vi "byte available write serial.vi"(11 "resourceId":i32) -> (2 "byte available":i32, 3 "resourceId out":i32)   [LabVIEW 2010, in "libcommon_serial.lvlib"]
doc: "int byte_available_write_serial(pserial_handle_t h);"
uses:
  <userlib>/libcommon_serial/libcommon_serial.lvlib
  <userlib>/libcommon_serial/libcommon_serial.so
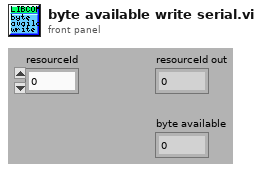
[diagram p1: front panel]
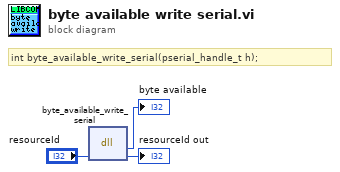
[diagram p0: block diagram]
diagram:
  # "int byte_available_write_serial(pserial_handle_t h);"
  n1 = dll-call lib="usr/local/natinst/LabVIEW-2010/user.lib/libcommon_serial/libcommon_serial.*" fn="byte_available_write_serial"("resourceId"="resourceId") -> (→"byte available":i32, "resourceId"=→"resourceId out":i32)  [unwired: 3 in, 2 out]
